vi "ConvertStringArrayToBoolArray.vi"(11 "String Array":string[](array[string])) -> (3 "Boolean Array":bool[](array[boolean]))   [LabVIEW 2012]
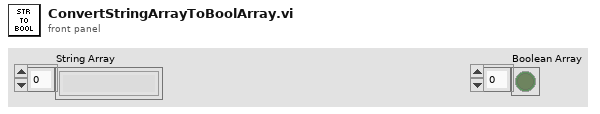
[diagram p1: front panel]
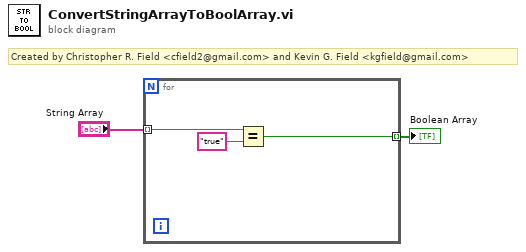
[diagram p0: block diagram]
diagram:
  # "Created by Christopher R. Field <cfield2@gmail.com> and Kevin G. Field <kgfield@gmail.com>"
  n1 = for {
    tunnel: "String Array" -> [w5] mode=indexing
    tunnel: [w3] -> w1 mode=indexing
    n2 = Equal?(x=w5, y="true") -> (x = y?=w3:bool)
  }
  "Boolean Array" <- w1
